vi "NML Data Acquisition V1.00.vi"() -> ()   [LabVIEW 2024]
doc: "This VI is designed to scan data each time the the trigger channel changes by an amount ? trigger. The first data column is converted to tesla using the magnet ID (or 'None' for volts).\nScott Hannahs, NHMFL - FSU, Mar 1996"
uses:
  Globals and TypeDefs/Global Varibal Control.vi
  xwei previous work/CCD Project/Subroutines/ExperimentLogGlobal.vi
  Sub VIs/McP Parameter.ctl
panel:
  in  "Trace\nHolders":u8=7 max=9 step=1
  out "McP Scan Parameter":T1={"McP on?"=TRUE, "Wait"=0.0, "X-Axis Unit String"="", "Data Format"=0, "Scanning Pattern:"=0, "Spex on?"=TRUE} {"Scanning Pattern:" items=["Uniform Points ", "User Defined Point Pattern ", "Time-Drive"]; "Data Format" items=["Original", "1024rows X 2cloumns", "Future Use"]; "Wait" format="%.2f"}
  in  "Setup":bool
  in  "SetDirectory?":bool
  in  "Current Path":path=path "/DATA/test"
  out "Current Path indicator":path=path "/DATA/test"
  in  "MainStop":bool
  in  "stop":bool
  in  "Display?":bool[](array[boolean])=[TRUE, FALSE, FALSE, FALSE, FALSE, FALSE, FALSE, FALSE, FALSE, FALSE, FALSE, FALSE, FALSE, FALSE, FALSE]
  out "# of columns":i32=1
  out "Index":i32=11
  out "Data Array":dbl[][](array[numeric])=[[1400.000573621509], [1400.000573621509], [1400.000573621509], [1400.000573621509], [1400.000573621509], [1400.000573621509], [1400.000573621509], [1400.000573621509], [1400.000573621509], [1400.000573621509], [1400.000573621509], [nan], [nan], [nan], [nan], [nan], [nan], [nan], [nan], [nan], [nan], [nan], [nan], [nan], [nan], [nan], [nan], [nan], [nan], [nan], [nan], [nan], [nan], [nan], [nan], [nan], [nan], [nan], [nan], [nan], [nan], [nan], [nan], [nan], [nan], [nan], [nan], [nan], [nan], [nan], [nan], [nan], [nan], [nan], [nan], [nan], [nan], [nan], [nan], [nan], [nan], [nan], [nan], [nan], [nan], [nan], [nan], [nan], [nan], [nan], [nan], [nan], [nan], [nan], [nan], [nan], [nan], [nan], [nan], [nan], [nan], [nan], [nan], [nan], [nan], [nan], [nan], [nan], [nan], [nan], [nan], [nan], [nan], [nan], [nan], [nan], [nan], [nan], [nan], [nan], [nan], [nan], [nan], [nan], [nan], [nan], [nan], [nan], [nan], [nan], [nan], [nan], [nan], [nan], [nan], [nan], [nan], [nan], [nan], [nan], [nan], [nan], [nan], [nan], [nan], [nan], [nan], [nan], [nan], [nan], [nan], [nan], [nan], [nan], [nan], [nan], [nan], [nan], [nan], [nan], [nan], [nan], [nan], [nan], [nan], [nan], [nan], [nan], [nan], [nan], [nan], [nan], [nan], [nan], [nan], [nan], [nan], [nan], [nan], [nan], [nan], [nan], [nan], [nan], [nan], [nan], [nan], [nan], [nan], [nan], [nan], [nan], [nan], [nan], [nan], [nan], [nan], [nan], [nan], [nan], [nan], [nan], [nan], [nan], [nan], [nan], [nan], [nan], [nan], [nan], [nan], [nan], [nan], [nan], [nan], [nan], [nan], [nan], [nan], [nan], [nan], [nan], [nan], [nan], [nan], [nan], [nan], [nan], [nan], [nan], [nan], [nan], [nan], [nan], [nan], [nan], [nan], [nan], [nan], [nan], [nan], [nan], [nan], [nan], [nan], [nan], [nan], [nan], [nan], [nan], [nan], [nan], [nan], [nan], [nan], [nan], [nan], [nan], [nan], [nan], [nan], [nan], [nan], [nan], [nan], [nan], [nan], [nan], [nan], [nan], [nan], [nan], [nan], [nan], [nan], [nan], [nan], [nan], [nan], [nan], [nan], [nan], [nan], [nan], [nan], [nan], [nan], [nan], [nan], [nan], [nan], [nan], [nan], [nan], [nan], [nan], [nan], [nan], [nan], [nan], [nan], [nan], [nan], [nan], [nan], [nan], [nan], [nan], [nan], [nan], [nan], [nan], [nan], [nan], [nan], [nan], [nan], [nan], [nan], [nan], [nan], [nan], [nan], [nan], [nan], [nan], [nan], [nan], [nan], [nan], [nan], [nan], [nan], [nan], [nan], [nan], [nan], [nan], [nan], [nan], [nan], [nan], [nan], [nan], [nan], [nan], [nan], [nan], [nan], [nan], [nan], [nan], [nan], [nan], [nan], [nan], [nan], [nan], [nan], [nan], [nan], [nan], [nan], [nan], [nan], [nan], [nan], [nan], [nan], [nan], [nan], [nan], [nan], [nan], [nan], [nan], [nan], [nan], [nan], [nan], [nan], [nan], [nan], [nan], [nan], [nan], [nan], [nan], [nan], [nan], [nan], [nan], [nan], [nan], [nan], [nan], [nan], [nan], [nan], [nan], [nan], [nan], [nan], [nan], [nan], [nan], [nan], [nan], [nan], [nan], [nan], [nan], [nan], [nan], [nan], [nan], [nan], [nan], [nan], [nan], [nan], [nan], [nan], [nan], [nan], [nan], [nan], [nan], [nan], [nan], [nan], [nan], [nan], [nan], [nan], [nan], [nan], [nan], [nan], [nan], [nan], [nan], [nan], [nan], [nan], [nan], [nan], [nan], [nan], [nan], [nan], [nan], [nan], [nan], [nan], [nan], [nan], [nan], [nan], [nan], [nan], [nan], [nan], [nan], [nan], [nan], [nan], [nan], [nan], [nan], [nan], [nan], [nan], [nan], [nan], [nan], [nan], [nan], [nan], [nan], [nan], [nan], [nan], [nan], [nan], [nan], [nan], [nan], [nan], [nan], [nan], [nan], [nan], [nan], [nan], [nan], [nan], [nan], [nan], [nan], [nan], [nan], [nan], [nan], [nan], [nan], [nan], [nan], [nan], [nan], [nan], [nan], [nan], [nan], [nan], [nan], [nan], [nan], [nan], [nan], [nan], [nan], [nan], [nan], [nan], [nan], [nan], [nan], [nan], [nan], [nan], [nan], [nan], [nan], [nan], [nan], [nan], [nan], [nan], [nan], [nan], [nan], [nan], [nan], [nan], [nan], [nan], [nan], [nan], [nan], [nan], [nan], [nan], [nan], [nan], [nan], [nan], [nan], [nan], [nan], [nan], [nan], [nan], [nan], [nan], [nan], [nan], [nan], [nan], [nan], [nan], [nan], [nan], [nan], [nan], [nan], [nan], [nan], [nan], [nan], [nan], [nan], [nan], [nan], [nan], [nan], [nan], [nan], [nan], [nan], [nan], [nan], [nan], [nan], [nan], [nan], [nan], [nan], [nan], [nan], [nan], [nan], [nan], [nan], [nan], [nan], [nan], [nan], [nan], [nan], [nan], [nan], [nan], [nan], [nan], [nan], [nan], [nan], [nan], [nan], [nan], [nan], [nan], [nan], [nan], [nan], [nan], [nan], [nan], [nan], [nan], [nan], [nan], [nan], [nan], [nan], [nan], [nan], [nan], [nan], [nan], [nan], [nan], [nan], [nan], [nan], [nan], [nan], [nan], [nan], [nan], [nan], [nan], [nan], [nan], [nan], [nan], [nan], [nan], [nan], [nan], [nan], [nan], [nan], [nan], [nan], [nan], [nan], [nan], [nan], [nan], [nan], [nan], [nan], [nan], [nan], [nan], [nan], [nan], [nan], [nan], [nan], [nan], [nan], [nan], [nan], [nan], [nan], [nan], [nan], [nan], [nan], [nan], [nan], [nan], [nan], [nan], [nan], [nan], [nan], [nan], [nan], [nan], [nan], [nan], [nan], [nan], [nan], [nan], [nan], [nan], [nan], [nan], [nan], [nan], [nan], [nan], [nan], [nan], [nan], [nan], [nan], [nan], [nan], [nan], [nan], [nan], [nan], [nan], [nan], [nan], [nan], [nan], [nan], [nan], [nan], [nan], [nan], [nan], [nan], [nan], [nan], [nan], [nan], [nan], [nan], [nan], [nan], [nan], [nan], [nan], [nan], [nan], [nan], [nan], [nan], [nan], [nan], [nan], [nan], [nan], [nan], [nan], [nan], [nan], [nan], [nan], [nan], [nan], [nan], [nan], [nan], [nan], [nan], [nan], [nan], [nan], [nan], [nan], [nan], [nan], [nan], [nan], [nan], [nan], [nan], [nan], [nan], [nan], [nan], [nan], [nan], [nan], [nan], [nan], [nan], [nan], [nan], [nan], [nan], [nan], [nan], [nan], [nan], [nan], [nan], [nan], [nan], [nan], [nan], [nan], [nan], [nan], [nan], [nan], [nan], [nan], [nan], [nan], [nan], [nan], [nan], [nan], [nan], [nan], [nan], [nan], [nan], [nan], [nan], [nan], [nan], [nan], [nan], [nan], [nan], [nan], [nan], [nan], [nan], [nan], [nan], [nan], [nan], [nan], [nan], [nan], [nan], [nan], [nan], [nan], [nan], [nan], [nan], [nan], [nan], [nan], [nan], [nan], [nan], [nan], [nan], [nan], [nan], [nan], [nan], [nan], [nan], [nan], [nan], [nan], [nan], [nan], [nan], [nan], [nan], [nan], [nan], [nan], [nan], [nan], [nan], [nan], [nan], [nan], [nan], [nan], [nan], [nan], [nan], [nan], [nan], [nan], [nan], [nan], [nan], [nan], [nan], [nan], [nan], [nan], [nan], [nan], [nan], [nan], [nan], [nan], [nan], [nan], [nan], [nan], [nan], [nan], [nan], [nan], [nan], [nan], [nan], [nan], [nan], [nan], [nan], [nan], [nan], [nan], [nan], [nan], [nan], [nan], [nan], [nan], [nan], [nan], [nan], [nan], [nan], [nan], [nan], [nan], [nan], [nan], [nan], [nan], [nan], [nan], [nan], [nan], [nan], [nan], [nan], [nan], [nan], [nan], [nan], [nan], [nan], [nan], [nan], [nan], [nan], [nan], [nan], [nan], [nan], [nan], [nan], [nan], [nan], [nan], [nan], [nan], [nan], [nan], [nan], [nan], [nan], [nan], [nan], [nan], [nan], [nan], [nan], [nan], [nan], [nan], [nan], [nan], [nan], [nan], [nan], [nan], [nan], [nan], [nan], [nan], [nan], [nan], [nan], [nan], [nan], [nan], [nan], [nan], [nan], [nan], [nan], [nan], [nan], [nan], [nan], [nan], [nan], [nan], [nan], [nan], [nan], [nan], [nan], [nan], [nan], [nan], [nan], [nan], [nan], [nan], [nan], [nan], [nan], [nan], [nan], [nan], [nan], [nan], [nan], [nan], [nan], [nan], [nan], [nan], [nan], [nan], [nan], [nan], [nan]] format="%.2f"
  in  "Print":bool
  out "X-Axis Label":string="nm"
  in  "Column Headings":string[](array[string])=["nm"]
  in  "Scale Factors":dbl[](array[numeric])=[1.0, 1.0, 1.0, 1.0, 1.0, 1.0, 1.0, 1.0, 1.0, 1.0, 1.0, 1.0, 1.0, 1.0, 1.0, 1.0, 1.0, 1.0, 1.0] format="%.3e"
  in  "Comments":string="This data's for you!\nType \u0011-H to get a help window for the various controls."
  in  "Monopolar\n\n\n\nBipolar":bool
  in  "Points Averaged":i32=128 min=3 max=32000
  out "Mode Indicator":string="Standby"
  in  "User Name":string="Conan The Scientist"
  in  "File Name":string="MyData.035"
  in  "TEST\nGPIB":bool
  in  "New/Stop":bool caption="Measurements"
  in  "X-Axis":i32(ring)=1 items=["Point #", "nm", "va1", "va1a", "va1b", "va1c", "va1d", "va1e", "va1f", "va1g", "va1h"]
  in  "Pause":bool=TRUE
  out "Data Plot":cluster{dbl[], dbl[]}[](graph)=[{[600.0, 601.0, 602.0, 603.0, 604.0, 605.0, 606.0, 607.0, 608.0, 609.0, 610.0, 611.0, 612.0, 613.0, 614.0, 615.0], [16666.666666666668, 16638.935108153077, 16611.295681063122, 16583.74792703151, 16556.29139072848, 16528.92561983471, 16501.6501650165, 16474.464579901152, 16447.36842105263, 16420.361247947454, 16393.44262295082, 16366.612111292963, 16339.869281045752, 16313.21370309951, 16286.644951140066, 16260.162601626016]}, {[600.0, 601.0, 602.0, 603.0, 604.0, 605.0, 606.0, 607.0, 608.0, 609.0, 610.0, 611.0, 612.0, 613.0, 614.0, 615.0], [2066.4040597731346, 2062.9657834673553, 2059.538930006446, 2056.123442560333, 2052.719264675299, 2049.326340270877, 2045.9446136367667, 2042.5740294297868, 2039.2145326708562, 2035.8660687420045, 2032.5285833834112, 2029.202022690476, 2025.8863331109162, 2022.5814614418935, 2019.2873548271675, 2016.0039607542776]}, {[600.0, 601.0, 602.0, 603.0, 604.0, 605.0, 606.0, 607.0, 608.0, 609.0, 610.0, 611.0, 612.0, 613.0, 614.0, 615.0], [0.0, 2.621, 5.119, 7.622, 10.12, 13.317, 16.011, 18.961, 21.524, 24.023, 26.519, 29.119, 31.62, 34.113, 36.621, 39.119]}, {[600.0, 601.0, 602.0, 603.0, 604.0, 605.0, 606.0, 607.0, 608.0, 609.0, 610.0, 611.0, 612.0, 613.0, 614.0, 615.0], [-9.447669, -9.4476764, -9.4476628, -9.447664, -9.4476628, -9.4476838, -9.4476677, -9.4476714, -9.4476714, -9.4476714, -9.4476788, -9.4476788, -9.4476677, -9.4476665, -9.4476727, -9.4476579]}]
  in  "CHANNEL & RANGE SELECTOR":T2 {"0" scale=0.0..4.0; "7" scale=0.0..4.0; "6" scale=0.0..4.0; "5" scale=0.0..4.0; "4" scale=0.0..4.0; "3" scale=0.0..4.0; "2" scale=0.0..4.0; "1" scale=0.0..4.0}
  in  "Æ Trigger":dbl min=0.0 format="%.3f"
  in  "Trigger Column":i32(ring)=1 items=["Time", "nm", "va1", "va1a", "va1b", "va1c", "va1d", "va1e", "va1f", "va1g", "va1h"]
  out "Data Record":string="   10\t  1.400E+3"
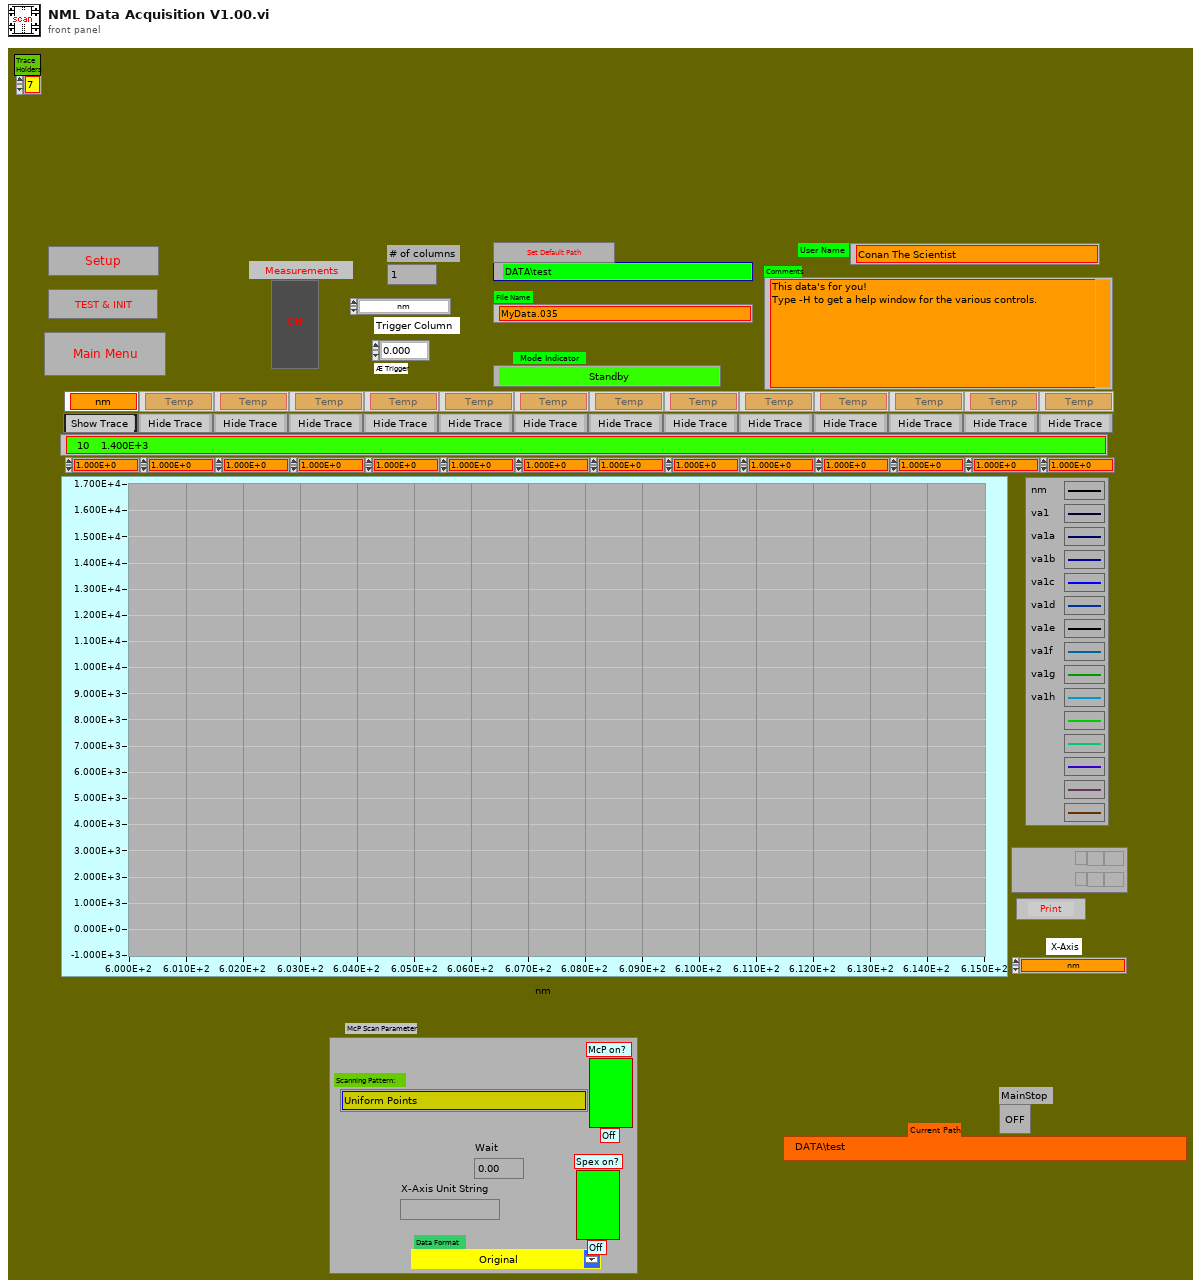
[diagram p1: front panel]
types:
  T1 = typedef "McP Parameter.ctl" = cluster{"McP on?":bool, "Wait":dbl, "X-Axis Unit String":string, "Data Format":u8, "Scanning Pattern:":u32, "Spex on?":bool}
  T2 = cluster{"0":i16, "1":i16, "2":i16, "3":i16, "4":i16, "5":i16, "6":i16, "7":i16}
  T3 = enum32{"existing file", "new file", "new or existing file", "existing dir", "new dir", "new or existing dir", "existing file (use LLBs)", "new file (use LLBs)", "new or existing file (use LLBs)", "new or existing file or directory (use LLBs)", "existing dir (use LLBs)", "new dir (use LLBs)", "new or existing dir (use LLBs)", "existing file or dir", "new file or dir", "new or existing file or dir", "existing file or dir (use LLBs)", "new file or dir (use LLBs)"}
  T4 = cluster{"top":i16, "left":i16, "bottom":i16, "right":i16}
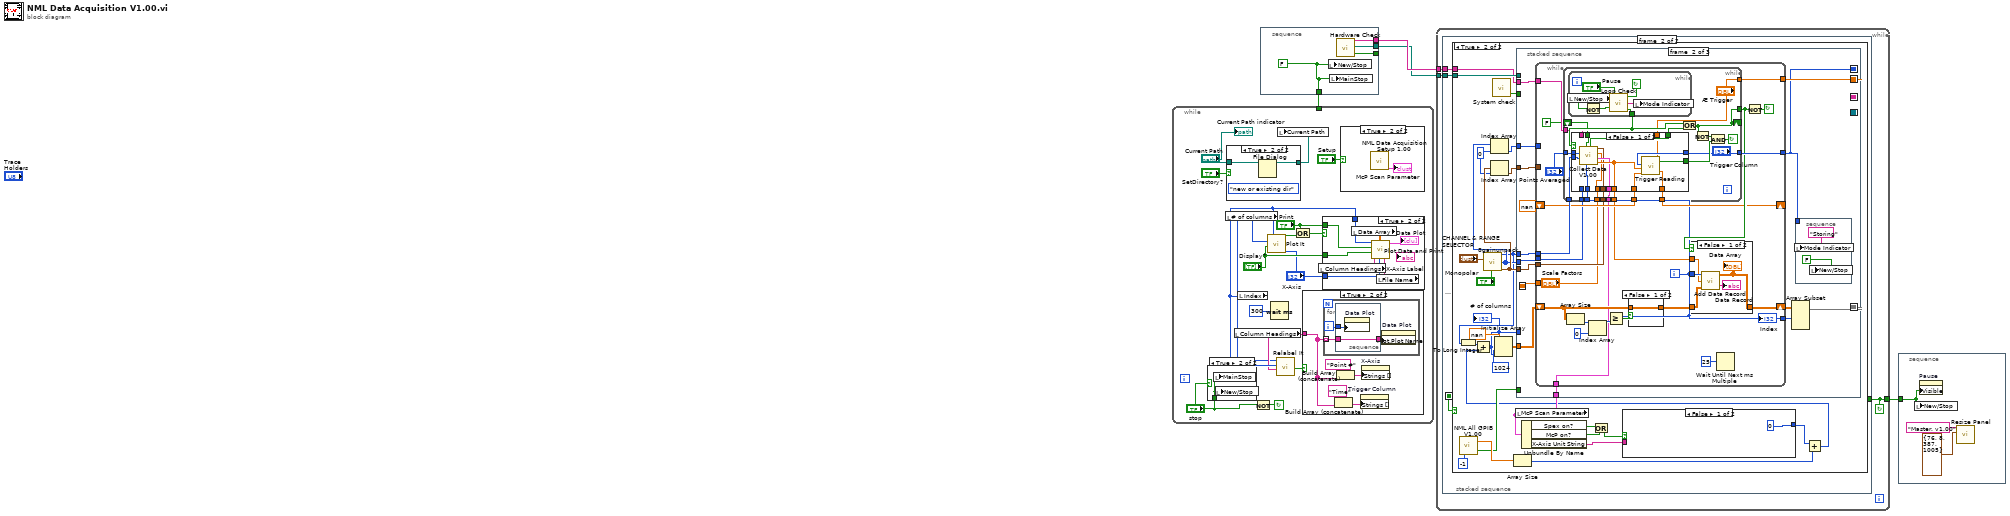
[diagram p0: block diagram]
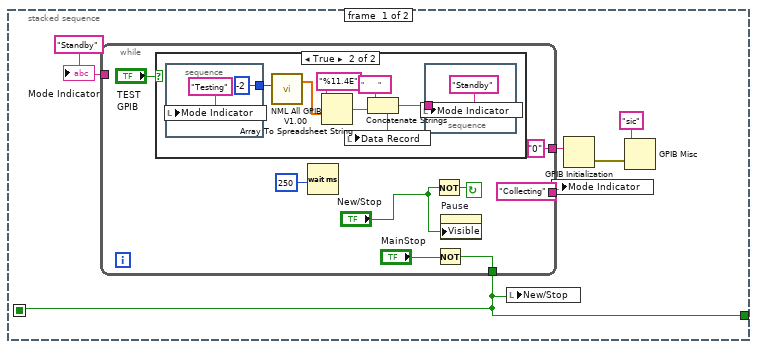
[diagram p2: hidden frame]
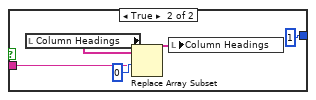
[diagram p5: hidden frame]
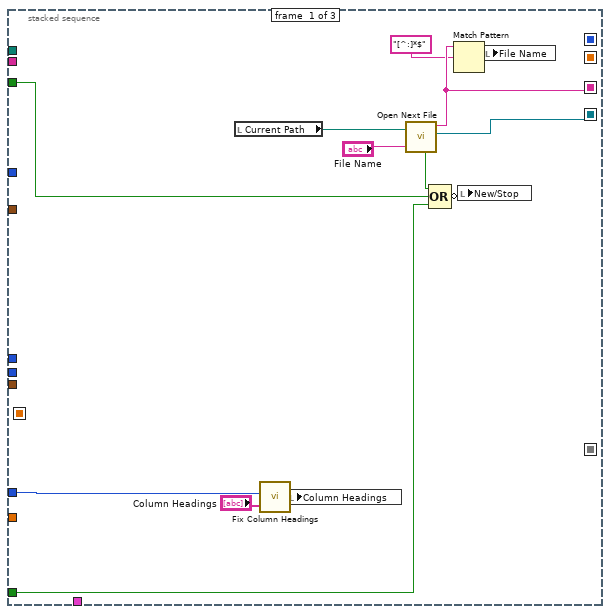
[diagram p6: hidden frame]
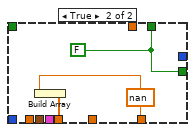
[diagram p7: hidden frame]
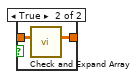
[diagram p9: hidden frame]
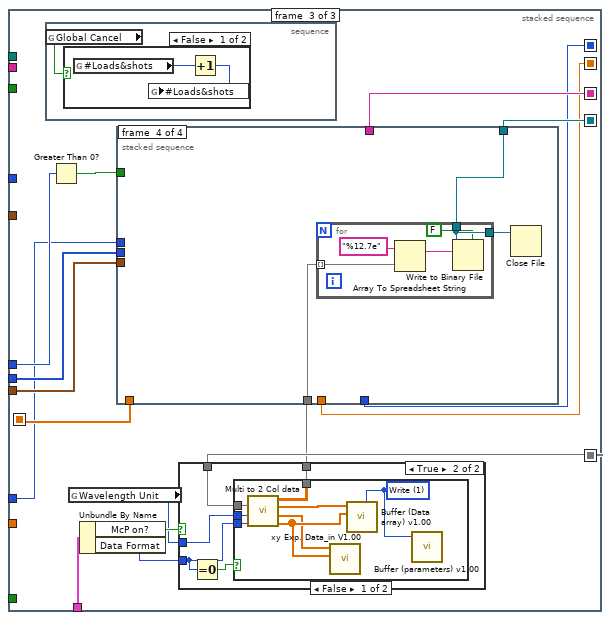
[diagram p10: hidden frame]
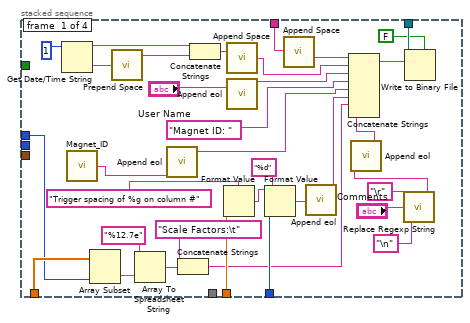
[diagram p14: hidden frame]
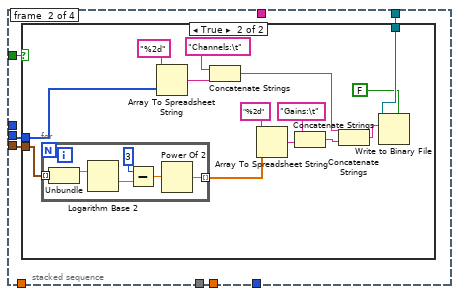
[diagram p15: hidden frame]
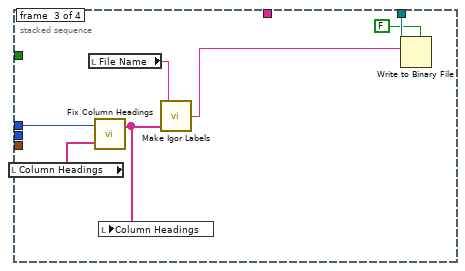
[diagram p17: hidden frame]
diagram:
  n1 = stacked-sequence {
    tunnel: [w8] -> w3
    tunnel: [w7] -> _
    tunnel: [w6] -> w4
    tunnel: [w5] -> w1
    frame #0 {
      w5 = FALSE ("New/Stop")
      n2 = local write "New/Stop"(w5) -> ()
      n3 = local write "MainStop"(w5) -> ()
      n4 = call "Hardware Check.vi"() -> ("Data Acq Device"=w6:string, "Data Directory Path"=w8:path, "Has A/D board"=w7:bool)  [unwired: 1 in]
    }
  }
  n5 = while {
    tunnel: w1 -> [_]
    stop <- w14 continue-if-true
    n6 = case shown="True" "stop" {
      tunnel: "stop" -> [_ w25]
      frame False {
      }
      frame True {
        n7 = local write "MainStop"(w25) -> ()
        n8 = local write "New/Stop"(w25) -> ()
      }
    }
    n9 = local read "# of columns"() -> (w23:i32)
    n10 = case shown="True" "SetDirectory?" {
      tunnel: [w27 w28] -> w11
      tunnel: "Current Path" -> [w27 w29]
      frame False {
      }
      frame True {
        (unwired) T3."new or existing dir" ("select mode (2)")
        n11 = File Dialog(11:w29) -> (3:w28:path)  [unwired: 6 in, 3 out]
      }
    }
    n12 = local read "Column Headings"() -> (w20:string[])
    n13 = local read "Index"() -> (w15:i32)
    n14 = Not(x="stop") -> (.not. x?=w14:bool)
    n15 = call "Plot It.vi"("X-Axis"="X-Axis", "Display?"="Display?", "# of columns"=w23, "Index"=w15) -> (0:w17:bool)
    n16 = Wait (ms)(milliseconds to wait=u32 300) -> ()  [unwired: 1 out]
    n17 = call "Relabel It.vi"("Index"=w15, "# of columns"=w23, "Column Headings"=w20) -> (5:w19:bool)  [unwired: 2 in]
    n18 = local write "Current Path"(w11) -> ()
    n19 = Or(x="Print", y=w17) -> (x .or. y?=w18:bool)
    n20 = case shown="True" w19 {
      tunnel: w20 -> [_ w34]
      frame False {
      }
      frame True {
        n21 = for {
          tunnel: w34 -> [w36] mode=indexing
          i -> [w37]
          n22 = stacked-sequence {
            tunnel: w37 -> [w39]
            tunnel: [w38] -> w35
            tunnel: w36 -> [w38]
            frame #0 {
              n23 = property on="Data Plot" class="XYGraph (strict)"("Active Plot"=w39) -> ()  [unwired: 2 in, 2 out]
            }
          }
          n24 = property on="Data Plot" class="XYGraph (strict)"("Plot.Plot Name"=w35) -> ()  [unwired: 2 in, 2 out]
        }
        n25 = Build Array (concatenate)("Time", w34) -> (w33:string[])
        n26 = Build Array (concatenate)("Point #", w34) -> (w31:string[])
        n27 = property on="Trigger Column" class="Ring (strict)"("Strings []"=w33) -> ()  [unwired: 2 in, 2 out]
        n28 = property on="X-Axis" class="Ring (strict)"("Strings []"=w31) -> ()  [unwired: 2 in, 2 out]
      }
    }
    n29 = case shown="True" w18 {
      tunnel: "Display?" -> [_ w47]
      tunnel: w15 -> [_ w46]
      tunnel: "X-Axis" -> [_ w41]
      tunnel: "Print" -> [_ w40]
      frame False {
      }
      frame True {
        n30 = local read "Column Headings"() -> (w42:string[])
        n31 = local read "Data Array"() -> (w43:dbl[][])
        n32 = local read "File Name"() -> (w45:string)
        n33 = call "Plot Data and Print.vi"("File:"=w45, "x axis column"=w41, "Data"=w43, "Col heading"=w42, "Display/hide"=w47, "Print"=w40, "Index"=w46) -> ("Data Plot"=→"Data Plot":cluster{dbl[], dbl[]}[])  [unwired: 2 in]
      }
    }
    n34 = case shown="True" "Setup" {
      frame False {
      }
      frame True {
        n35 = call "NML Data Acquisition Setup 1.00.vi"() -> ("McP Scan Parameter"=→"McP Scan Parameter":T1)  [unwired: 8 in, 1 out]
      }
    }
    "Current Path indicator" <- "Current Path"
  }
  n36 = while {
    tunnel: [w48] -> w2
    tunnel: w4 -> [w49]
    tunnel: w3 -> [w50]
    stop <- w48 continue-if-true
    n37 = stacked-sequence {
      seq-local: [w51 _] -> [_ w74]
      tunnel: w50 -> [_ w76]
      tunnel: w49 -> [_ w75]
      tunnel: [w51 _] -> w48
      frame #0 {
        w54 = "Standby"
        n38 = while {
          tunnel: [w57] -> w51
          tunnel: ["Collecting"] -> w52
          tunnel: w54 -> [_]
          tunnel: ["0"] -> w53
          stop <- w64 continue-if-true
          n39 = case shown="True" "TEST\nGPIB" {
            frame False {
            }
            frame True {
              n40 = stacked-sequence {
                tunnel: [-2] -> w65
                frame #0 {
                  n41 = local write "Mode Indicator"("Testing") -> ()
                }
              }
              n42 = call "NML All GPIB V1.00.vi"("Point #"=w65) -> ("GPIB Data Out"=w70:dbl[])  [unwired: 1 out]
              n43 = Array To Spreadsheet String(array=w70, 3:"%11.4E") -> (spreadsheet string=w67:string)  [unwired: 1 in]
              n44 = Concatenate Strings("       ", w67) -> (w68:string)
              n45 = local write "Data Record"(w68) -> ()
              n46 = stacked-sequence {
                tunnel: w68 -> [_]
                frame #0 {
                  n47 = local write "Mode Indicator"("Standby") -> ()
                }
              }
            }
          }
          n48 = Wait (ms)(milliseconds to wait=u32 250) -> ()  [unwired: 1 out]
          n49 = Not(x="New/Stop") -> (.not. x?=w64:bool)
          n50 = Not(x="MainStop") -> (.not. x?=w57:bool)
          n51 = property on="Pause" class="Bool (strict)"("Visible"="New/Stop") -> ()  [unwired: 2 in, 2 out]
        }
        n52 = local write "New/Stop"(w51) -> ()
        n53 = local write "Mode Indicator"(w52) -> ()
        n54 = GPIB Initialization(6:w53) -> (0:w55:errorcluster)  [unwired: 6 in]
        n55 = GPIB Misc(0:"sic", 1:w55) -> ()  [unwired: 3 out]
        "Mode Indicator" <- w54
      }
      frame #1 {
        n56 = case shown="True" w74 {
          tunnel: w76 -> [_ w92]
          tunnel: w75 -> [_ w91]
          frame False {
          }
          frame True {
            w98 = 0
            n57 = call "NML All GPIB V1.00.vi"("Point #"=-1) -> ("GPIB Data Out"=w96:dbl[], "Stop Out"=w85:bool)
            n58 = call "8gainunpack.vi"("GAIN & CHANNEL SELECTOR"="CHANNEL & RANGE SELECTOR", "Monopolar"="Monopolar\n\n\n\nBipolar") -> ("Number of channels"=w88:i32, "channels (0)"=w99:i32[], "Input Limits"=w103:cluster{"High Limit":dbl, "Low Limit":dbl}[])
            n59 = To Long Integer(number=w88) -> (32bit integer=w102:i32)
            n60 = Index Array(array=w99, index=w98) -> (element=w101:i32)
            n61 = Index Array(array=w103, index=w98) -> (element=w100:cluster{"High Limit":dbl, "Low Limit":dbl})
            n62 = call "System check.vi"() -> ("Abort"=w86:bool)  [unwired: 3 in]
            n63 = Array Size(array=w96) -> (size(s)=w83:i32)
            n64 = local read "McP Scan Parameter"() -> (w84:T1)
            n65 = Unbundle By Name(w84) -> ("Spex on?"=w79:bool, "McP on?"=w77:bool, "X-Axis Unit String"=w80:string)
            n66 = Or(x=w79, y=w77) -> (x .or. y?=w78:bool)
            n67 = case shown="False" w78 {
              tunnel: [0 1] -> w81
              tunnel: w80 -> [_ w105]
              frame False {
              }
              frame True {
                n68 = local read "Column Headings"() -> (w108:string[])
                n69 = Replace Array Subset(array=w108, new element=w105, index=0 ("Index")) -> (w107:string[])
                n70 = local write "Column Headings"(w107) -> ()
              }
            }
            n71 = Add(x=w81, y=w83) -> (x+y=w82:i32)
            n72 = Add(x=w102, y=w82) -> (x+y=w87:i32)
            "# of columns" <- w87
            n73 = Initialize Array(nan, 1024, w87) -> (w97:dbl[][])
            n74 = stacked-sequence "file Name" {
              seq-local: [_ w124 _] -> [_ _ w226]
              seq-local: [_ w130 _] -> [_ _ w220]
              seq-local: [_ w137 _] -> [_ _ w227]
              seq-local: [w122 _ _] -> [_ _ w231]
              seq-local: [w121 _ _] -> [_ _ w228]
              seq-local: [_ w128 _] -> [_ _ w223]
              tunnel: w97 -> [_ w125 _]
              tunnel: w91 -> [_ w131 _]
              tunnel: w101 -> [_ w132 _]
              tunnel: w100 -> [_ w133 _]
              tunnel: w103 -> [_ w134 w229]
              tunnel: w99 -> [_ w135 w230]
              tunnel: w88 -> [_ w136 w224]
              tunnel: w87 -> [w116 _ w222]
              tunnel: w92 -> [_ _ _]
              tunnel: w86 -> [w112 _ _]
              tunnel: w85 -> [w111 _ _]
              tunnel: w84 -> [_ w123 w221]
              frame #0 {
                n75 = local read "Current Path"() -> (w110:path)
                n76 = call "Fix Column Headings.vi"("Column Headings"="Column Headings", "# Cols"=w116) -> ("Column Headings"=w115:string[])
                n77 = local write "Column Headings"(w115) -> ()
                n78 = call "Open Next File.vi"("Input File Pattern"="File Name", "Dir Path"=w110) -> ("File Ref Num"=w122:refnum<file>, "Output File Name"=w121:string, "Stop"=w113:bool)  [unwired: 1 in, 1 out]
                n79 = Compound Arithmetic op=OR(w113, w112, w111) -> (invert w114:bool)
                n80 = Match Pattern(string=w121, regular expression="[^:]*$") -> (match substring=w118:string)  [unwired: 1 in, 3 out]
                n81 = local write "New/Stop"(w114) -> ()
                n82 = local write "File Name"(w118) -> ()
              }
              frame #1 {
                n83 = while {
                  tunnel: w123 -> [w139]
                  tunnel: ["Scale Factors"] -> w128
                  tunnel: w133 -> [_]
                  tunnel: w134 -> [w145]
                  tunnel: w135 -> [w147]
                  tunnel: w136 -> [w154]
                  tunnel: w132 -> [_]
                  tunnel: [w160] -> w137
                  tunnel: w131 -> [w159]
                  tunnel: [w140] -> w126
                  tunnel: [w151] -> w124
                  shift-left: nan -> [w148]
                  shift-right: [w149] -> _
                  shift-left: w125 -> [w155]
                  shift-right: [w161] -> w127
                  i -> [w140]
                  stop <- w143 continue-if-true
                  n84 = while {
                    shift-left: FALSE -> [w163]
                    shift-right: [w162] -> _
                    tunnel: w159 -> [w178]
                    tunnel: [w162] -> w150
                    tunnel: ["Æ Trigger"] -> w160
                    tunnel: "Points Averaged" -> [w172]
                    tunnel: w154 -> [w173]
                    tunnel: ["Trigger Column"] -> w151
                    tunnel: w148 -> [w175]
                    tunnel: [w174] -> w149
                    tunnel: w140 -> [w171]
                    tunnel: w147 -> [w170]
                    tunnel: [w169] -> w146
                    tunnel: w139 -> [w168]
                    tunnel: w145 -> [w167]
                    tunnel: "Scale Factors" -> [w166]
                    stop <- w180 continue-if-true
                    n85 = while {
                      tunnel: [w185] -> w179
                      stop <- w186 continue-if-true
                      n86 = local read "New/Stop"() -> (w183:bool)
                      n87 = Not(x=w183) -> (.not. x?=w184:bool)
                      n88 = call "Loop Check.vi"("Pause"="Pause", "Stop"=w184) -> ("Pause"=w186:bool, "State"=w182:string, "ABORT"=w185:bool)
                      n89 = local write "Mode Indicator"(w182) -> ()
                    }
                    n90 = case shown="False" w179 {
                      tunnel: "Æ Trigger" -> [w190 _]
                      tunnel: w163 -> [w191 _]
                      tunnel: [w192 w204] -> w165
                      tunnel: w166 -> [w188 _]
                      tunnel: w167 -> [w193 _]
                      tunnel: w168 -> [w194 _]
                      tunnel: [w195 w202] -> w169
                      tunnel: w170 -> [_ _]
                      tunnel: w171 -> [w196 _]
                      tunnel: w172 -> [w197 _]
                      tunnel: w173 -> [w198 _]
                      tunnel: [w189 w203] -> w174
                      tunnel: w175 -> [w199 _]
                      tunnel: "Trigger Column" -> [w200 _]
                      tunnel: [w201 w204] -> w177
                      tunnel: w178 -> [_ _]
                      frame False {
                        n91 = call "Collect Data V1.00.vi"("McP Scan Parameter"=w194, "Scaling Factors"=w188, "input limits (no change)"=w193, "Point Number"=w196, "stop"=w191, "Number of Channels"=w198, "Number to Average"=w197) -> ("Output Data"=w195:dbl[], "Stop"=w192:bool)  [unwired: 2 in]
                        n92 = call "Trigger Reading.vi"("Old Trigger Value"=w199, "Current Values"=w195, "Trigger Column"=w200, "Æ Trigger Value"=w190) -> ("New Trigger Value"=w189:dbl, "Wait"=w201:bool)
                      }
                      frame True {
                        w204 = FALSE
                        w203 = nan
                        n93 = Build Array(w203) -> (w202:dbl[])
                      }
                    }
                    n94 = Or(x=w179, y=w165) -> (x .or. y?=w162:bool)
                    n95 = Not(x=w162) -> (.not. x?=w181:bool)
                    n96 = And(x=w181, y=w177) -> (x .and. y?=w180:bool)
                  }
                  n97 = Array Size(array=w155) -> (size(s)=w152:i32[])
                  n98 = Index Array(array=w152, index=0) -> (element=w158:i32)
                  n99 = Greater Or Equal?(x=w140, y=w158) -> (x >= y?=w156:bool)
                  n100 = case shown="False" w156 {
                    tunnel: [w211 w212] -> w153
                    tunnel: w155 -> [w211 w213]
                    frame False {
                    }
                    frame True {
                      n101 = call "Check and Expand Array.vi"(1:w213) -> (0:w212:dbl[][])
                    }
                  }
                  n102 = case shown="False" w150 {
                    tunnel: w146 -> [w206 _]
                    tunnel: [w205 w210] -> w161
                    tunnel: w140 -> [w209 _]
                    tunnel: w153 -> [w208 w210]
                    frame False {
                      n103 = call "Add Data Record.vi"("Data In"=w208, "Data to update"=w206, "Index"=w209) -> ("Data Display"=→"Data Record":string, "Data Out"=w205:dbl[][])  [unwired: 1 in]
                      "Data Array" <- w205
                    }
                    frame True {
                    }
                  }
                  n104 = Wait Until Next ms Multiple(millisecond multiple=u32 25) -> ()  [unwired: 1 out]
                  n105 = Not(x=w150) -> (.not. x?=w143:bool)
                  "Index" <- w140
                }
                n106 = Array Subset(array=w127, length (row)=w126) -> (w130:dbl[][])  [unwired: 3 in]
                n107 = stacked-sequence {
                  tunnel: w124 -> [_]
                  frame #0 {
                    n108 = local write "Mode Indicator"("Storing") -> ()
                    n109 = local write "New/Stop"(FALSE) -> ()
                  }
                }
              }
              frame #2 {
                n110 = stacked-sequence {
                  frame #0 {
                    n111 = global read "Global Varibal Control.vi" "Global Cancel"() -> (w232:bool)
                    n112 = case shown="False" w232 {
                      frame False {
                        n113 = global read "ExperimentLogGlobal.vi" "#Loads&shots"() -> (w234:u32)
                        n114 = Increment(x=w234) -> (x+1=w233:u32)
                        n115 = global write "ExperimentLogGlobal.vi" "#Loads&shots"(w233) -> ()
                      }
                      frame True {
                      }
                    }
                  }
                }
                n116 = Greater Than 0?(x=w224) -> (x > 0?=w225:bool)
                n117 = global read "Global Varibal Control.vi" "Wavelength Unit"() -> (w216:u8)
                n118 = Unbundle By Name(w221) -> ("McP on?"=w217:bool, "Data Format"=w218:u8)
                n119 = case shown="True" w217 {
                  tunnel: w220 -> [w235 w240]
                  tunnel: w216 -> [_ w239]
                  tunnel: w218 -> [_ w237]
                  tunnel: [w235 w238] -> w219
                  frame False {
                  }
                  frame True {
                    n120 = Equal To 0?(x=w237) -> (x = 0?=w236:bool)
                    n121 = case shown="False" w236 {
                      tunnel: w240 -> [w248 w249]
                      tunnel: w239 -> [w247 _]
                      tunnel: w237 -> [w246 _]
                      tunnel: [w245 w249] -> w238
                      frame False {
                        w244 = u16 1 items=["Read", "Write", "Initialize"] ("Read(0) or Write(1)")
                        n122 = call "Multi to 2 Col data.vi"("Data Format"=w246, "X-Axis Unit"=w247, "DataIn"=w248) -> ("Y output"=w242:dbl[], "X-Axis Output"=w241:dbl[], "X-Axis (nm) Output"=w243:dbl[], "DataOut"=w245:dbl[][])  [unwired: 3 in]
                        n123 = call "xy Exp. Data_in V1.00.vi"("X-axis row"=w241, "Data row"=w242) -> ()  [unwired: 3 in, 2 out]
                        n124 = call "Buffer (Data array) v1.00.vi"("Action"=w244, "Y Data In"=w242, "X Data In"=w243) -> ()  [unwired: 5 in, 4 out]
                        n125 = call "Buffer (parameters) v1.00.vi"("Action"=w244) -> ()  [unwired: 10 in, 5 out]
                      }
                      frame True {
                      }
                    }
                  }
                }
                n126 = stacked-sequence {
                  tunnel: w226 -> [w267 _ _ _]
                  tunnel: w227 -> [w270 _ _ _]
                  tunnel: w228 -> [w271 _ _ _]
                  tunnel: w219 -> [_ _ _ w317]
                  tunnel: w229 -> [_ w286 _ _]
                  tunnel: w230 -> [_ w287 _ _]
                  tunnel: w231 -> [w264 w288 w315 w318]
                  tunnel: w225 -> [_ w285 _ _]
                  tunnel: w223 -> [w257 _ _ _]
                  tunnel: w222 -> [w256 _ w313 _]
                  frame #0 {
                    n127 = Get Date/Time String(date format (0)=1) -> (date string=w276:string, time string=w274:string)  [unwired: 2 in]
                    n128 = call "Magnet_ID.vi"() -> ("Cell"=w251:string)
                    n129 = Array Subset(array=w257, length=w256) -> (w258:dbl[])  [unwired: 1 in]
                    n130 = call "Prepend Space.vi"("Input String"=w274) -> ("Space + Input String"=w275:string)
                    n131 = Array To Spreadsheet String(array=w258, 3:"%12.7e") -> (spreadsheet string=w262:string)  [unwired: 1 in]
                    n132 = call "Append eol.vi"("INPUT STRING"=w251) -> ("OUTPUT STRING (PLUS End of Line)"=w278:string)
                    n133 = Concatenate Strings("Scale Factors:\t", w262) -> (w260:string)
                    n134 = Concatenate Strings(w276, w275) -> (w277:string)
                    n135 = Format Value(format string="Trigger spacing of %g on column #", value (0)=w270) -> (output string=w269:string)  [unwired: 1 in]
                    n136 = call "Append Space.vi"("INPUT STRING"=w277) -> ("OUTPUT STRING (PLUS [SPACE])"=w281:string)
                    n137 = call "Append eol.vi"("INPUT STRING"="User Name") -> ("OUTPUT STRING (PLUS End of Line)"=w280:string)
                    n138 = Format Value(string ("")=w269, format string="%d", value (0)=w267) -> (output string=w268:string)
                    n139 = call "Append Space.vi"("INPUT STRING"=w271) -> ("OUTPUT STRING (PLUS [SPACE])"=w282:string)
                    n140 = call "Append eol.vi"("INPUT STRING"=w268) -> ("OUTPUT STRING (PLUS End of Line)"=w265:string)
                    n141 = call "Replace Regexp String.vi"("Search String"="\n", "Input String"="Comments", "Replacement String"="\r") -> ("Output String"=w255:string)
                    n142 = call "Append eol.vi"("INPUT STRING"=w255) -> ("OUTPUT STRING (PLUS End of Line)"=w259:string)
                    n143 = Concatenate Strings(w282, w281, w280, "Magnet ID: ", w278, w265, w260, w259) -> (w284:string)
                    n144 = Write to Binary File(file (use dialog)=w264, data=w284, 5:FALSE ("prepend array or string size? (T)")) -> ()  [unwired: 3 in, 3 out]
                  }
                  frame #1 {
                    n145 = case shown="True" w285 {
                      tunnel: w287 -> [_ w293]
                      tunnel: w286 -> [_ w291]
                      tunnel: w288 -> [_ w292]
                      frame False {
                      }
                      frame True {
                        n146 = for {
                          tunnel: w291 -> [w308] mode=indexing
                          tunnel: [w303] -> w290 mode=indexing
                          n147 = Unbundle(w308) -> ("High Limit"=w307:dbl)  [unwired: 1 out]
                          n148 = Logarithm Base 2(1:w307) -> (0:w306:dbl)
                          n149 = Subtract(x=3, y=w306) -> (x-y=w304:dbl)
                          n150 = Power Of 2(x=w304) -> (2^x=w303:dbl)
                        }
                        n151 = Array To Spreadsheet String(array=w293, 3:"%2d") -> (spreadsheet string=w294:string)  [unwired: 1 in]
                        n152 = Concatenate Strings("Channels:\t", w294) -> (w301:string)
                        n153 = Array To Spreadsheet String(array=w290, 3:"%2d") -> (spreadsheet string=w299:string)  [unwired: 1 in]
                        n154 = Concatenate Strings("Gains:\t", w299) -> (w302:string)
                        n155 = Concatenate Strings(w301, w302) -> (w297:string)
                        n156 = Write to Binary File(file (use dialog)=w292, data=w297, 5:FALSE ("prepend array or string size? (T)")) -> ()  [unwired: 3 in, 3 out]
                      }
                    }
                  }
                  frame #2 {
                    n157 = local read "Column Headings"() -> (w314:string[])
                    n158 = local read "File Name"() -> (w310:string)
                    n159 = call "Fix Column Headings.vi"("Column Headings"=w314, "# Cols"=w313) -> ("Column Headings"=w312:string[])
                    n160 = local write "Column Headings"(w312) -> ()
                    n161 = call "Make Igor Labels.vi"("Column Names"=w312, "File Name"=w310) -> ("Igor Column Headings"=w311:string)
                    n162 = Write to Binary File(file (use dialog)=w315, data=w311, 5:FALSE ("prepend array or string size? (T)")) -> ()  [unwired: 3 in, 3 out]
                  }
                  frame #3 {
                    n163 = for {
                      tunnel: w317 -> [w322] mode=indexing
                      tunnel: w318 -> [w320]
                      tunnel: [w320] -> w316
                      n164 = Array To Spreadsheet String(array=w322, 3:"%12.7e") -> (spreadsheet string=w321:string)  [unwired: 1 in]
                      n165 = Write to Binary File(file (use dialog)=w320, data=w321, 5:FALSE ("prepend array or string size? (T)")) -> ()  [unwired: 3 in, 3 out]
                    }
                    n166 = Close File(refnum=w316) -> ()  [unwired: 1 in, 2 out]
                  }
                }
              }
            }
          }
        }
      }
    }
  }
  n167 = stacked-sequence {
    tunnel: w2 -> [w326]
    frame #0 {
      n168 = local write "New/Stop"(w326) -> ()
      n169 = property on="Pause" class="Bool (strict)"("Visible"=w326) -> ()  [unwired: 2 in, 2 out]
      n170 = call <vilib>:"Resize Panel.vi"("panel location and size"=T4 {"top"=76, "left"=8, "bottom"=387, "right"=1005}, "VI name"="Master. v1.00") -> ()  [unwired: 9 in, 1 out]
    }
  }
